vi "runEventApp.vi"   [LabVIEW 2009, in "Events.lvlib"]
uses:
  Events.lvlib
  ScriptEvent.lvclass
  Sender/sender.lvclass
  Receiver/receiver.lvclass
  Event.lvclass
panel:
  # "runs script event app"
types:
  T1 = enum32{"Invalid", "Standard", "Closed", "Hidden", "Minimized", "Maximized"}
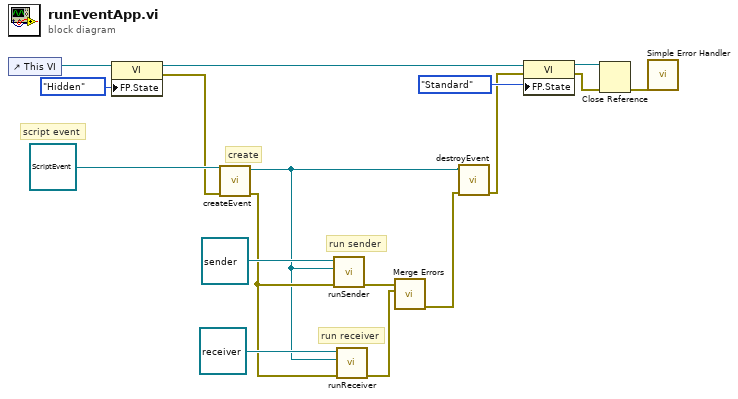
[diagram p0: block diagram]
diagram:
  # "run receiver"
  # "run sender"
  # "create"
  # "script event"
  n1 = control-ref of="This VI"() -> (w17:refnum<vi>)
  n2 = property class="VI"(reference=w17, "FP.State"=T1."Hidden" ("Front Panel Window:State")) -> (reference out=w5:refnum<vi>, error out=w14:errorcluster)  [unwired: 1 in]
  n3 = call "createEvent.vi"("error in (no error)"=w14, "Event in"=refnum<class "ScriptEvent.lvclass"> refnum ("ScriptEvent.lvclass")) -> ("error out"=w11:errorcluster, "Event out"=w7:refnum<class "ScriptEvent.lvclass">)  [unwired: 8 in]
  n4 = call "runSender.vi"("error in (no error)"=w11, "ScriptEvent"=w7, "sender in"=refnum<class "sender.lvclass"> refnum ("sender.lvclass")) -> ("error out"=w10:errorcluster)  [unwired: 7 in, 1 out]
  n5 = call "runReceiver.vi"("error in (no error)"=w11, "ScriptEvent"=w7, "receiver in"=refnum<class "receiver.lvclass"> refnum ("receiver.lvclass")) -> ("error out"=w9:errorcluster)  [unwired: 7 in, 1 out]
  n6 = call <vilib>:"Merge Errors.vi"("error in 2 (no error)"=w9, "error in 1 (no error)"=w10) -> ("error out"=w8:errorcluster)  [unwired: 5 in]
  n7 = call "destroyEvent.vi"("error in (no error)"=w8, "Event in"=w7) -> ("error out"=w4:errorcluster)  [unwired: 8 in, 1 out]
  n8 = property class="VI"(reference=w5, error in=w4, "FP.State"=T1."Standard" ("Front Panel Window:State")) -> (reference out=w2:refnum<vi>, error out=w3:errorcluster)
  n9 = Close Reference(reference=w2, error in (no error)=w3) -> (error out=w1:errorcluster)
  n10 = call <vilib>:"Simple Error Handler.vi"("error in (no error)"=w1) -> ()  [unwired: 4 in, 5 out]
